vi "CSMP-Broadcast.vi"(0 "State":string, 1 "Args":string, 2 "Source/target":string, 4 "Response For Message.’Error":errorcluster, 5 "Error In":errorcluster caption="error in (no error)", 8 "Module Name":string, 10 "Msg Type":T1=enum."Broadcast(-><status>)") -> (14 "State Out":string, 15 "Args Out":string, 16 "Source/target Out":string, 17 "Pre-State Out":string, 18 "Pre-Args Out":string, 19 "Error":errorcluster)   [LabVIEW 2017, in "Communicable State Machine.lvlib"]
doc: "### CSMP-Broadcast.vi\n\n-- <b>Controls</b> --\n- <b>state</b>:\n- <b>args</b>:\n- <b>source/target</b>:\n- <b>Module Name</b>:\n- <b>Msg Type</b>:\n\n-- <b>Indicators</b> --\n- <b>state out</b>:\n- <b>args out</b>:\n- <b>source/target out</b>:\n- <b>Pre-State out</b>:\n- <b>Pre-Args out</b>:\n- <b>error</b>:"
uses:
  Communicable State Machine.lvlib
  Typedef/_CSM_MSG_TYPE.ctl
  Typedef/_CSM Status Change Event Data.ctl
  Typedef/_Cross CSM State Data.ctl
  Typedef/_Cross CSM State Response.ctl
  Typedef/_CSM_Response Source Message.ctl
  AdvanceAPI/CSM - Make String Arguments Safe.vi
  Priority Queue/Enqueue Element.vi
  ChangeFlag/FlagInstance-CSMQ FGV.vi
  ChangeFlag/FlagInstance-Broadcast Cache.vi
  _Shared/Trim Single-line Text.vi
  AdvanceAPI/CSM - Keywords.vi
  ChangeFlag/ChangeFlag-Read.vi
  CSMQ/_CSMOFGV(lvlibp).vi
  FGV-BroadcastRegistry/FGV-BroadcastRegistry(lvlibp).vi
  BroadcastRegistry/HelperVI/Broadcast Item Key.vi
  ChangeFlag/ChangeFlagDB.vi
  AdvanceAPI/CSM - List Modules.vi
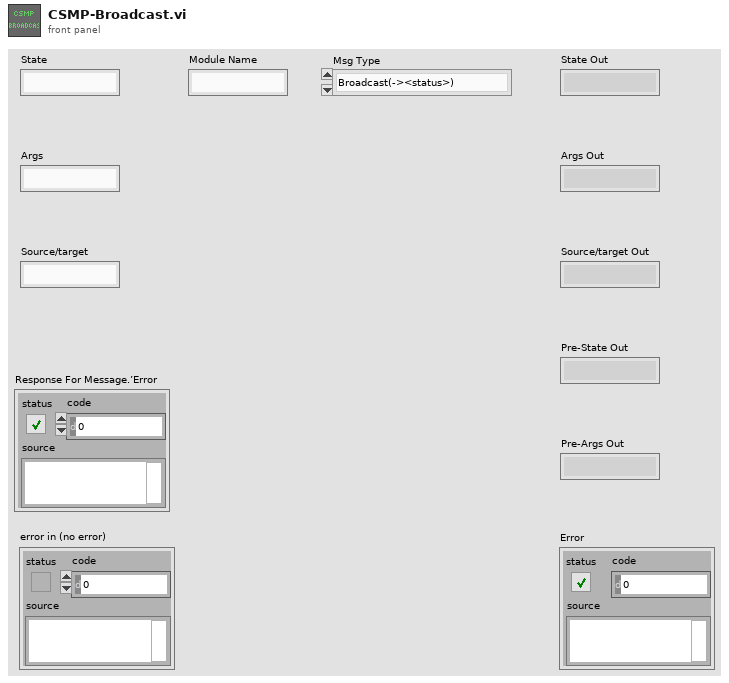
[diagram p1: front panel]
types:
  T1 = typedef "Communicable State Machine.lvlib/_CSM_MSG_TYPE.ctl" = enum16{"Sync Message(-@)", "Async Message(->)", "Async without Response(->|)", "Async Response", "Broadcast(-><all>)", "Broadcast(-><status>)", "Broadcast(-><interrupt>)", "Append to JKISM States", "Append to JKISM States(High Priority)", "Broadcast(-><state>)", "<None>"}
  T2 = typedef "Communicable State Machine.lvlib/_CSM Status Change Event Data.ctl" = cluster{"ModuleName":string, "Status":string, "Arguments":string}
  T3 = typedef "Communicable State Machine.lvlib/CSM - Broadcast Message Type.ctl" = enum16{"<Null>", "Status", "Interrupt"}
  T4 = cluster{"Target CSM":string, "Target State":string, "Register Type":T3}[]
  T5 = typedef "Communicable State Machine.lvlib/_Cross CSM State Data.ctl" = cluster{"Msg Type":T1, "state":string, "args":string, "source":string, "RespQ":refnum<queue>, "Response For Message":T6, "Target":string}
  T6 = typedef "Communicable State Machine.lvlib/_CSM_Response Source Message.ctl" = cluster{"‘State":string, "’Arguments":string, "’Error":errorcluster}
  T7 = typedef "Communicable State Machine.lvlib/_CSMObj.ctl" = cluster{"info":T8, "Refs":T10}
  T8 = typedef "Communicable State Machine.lvlib/_CSMObj-Info.ctl" = cluster{"Module Name":string, "Requested Name":string, "Group Name":string, "Mode":T9, "Allowed Messages":string[]}
  T9 = typedef "Communicable State Machine.lvlib/_CSM_MODE.ctl" = enum16{"Not Exist", "Stand Alone", "CSM", "Worker", "Worker Agent", "Chain Node", "Chain"}
  T10 = typedef "Communicable State Machine.lvlib/_CSMObj-Refs.ctl" = cluster{"WatchDogQ":refnum<queue>, "CSMDataDVR":refnum<data-value>, "Queue":T11, "GroupDataDVR":refnum<data-value>, "TagMap":refnum<data-value>, "ExitEvent":refnum<user-event>, "NewStateEvent":refnum<user-event>, "StatusEvent":refnum<user-event>, "InterruptEvent":refnum<user-event>}
  T11 = typedef "Communicable State Machine.lvlib/Priority Queue.ctl" = cluster{"HPriorityQ":refnum<queue>, "LowPriorityQ":refnum<queue>}
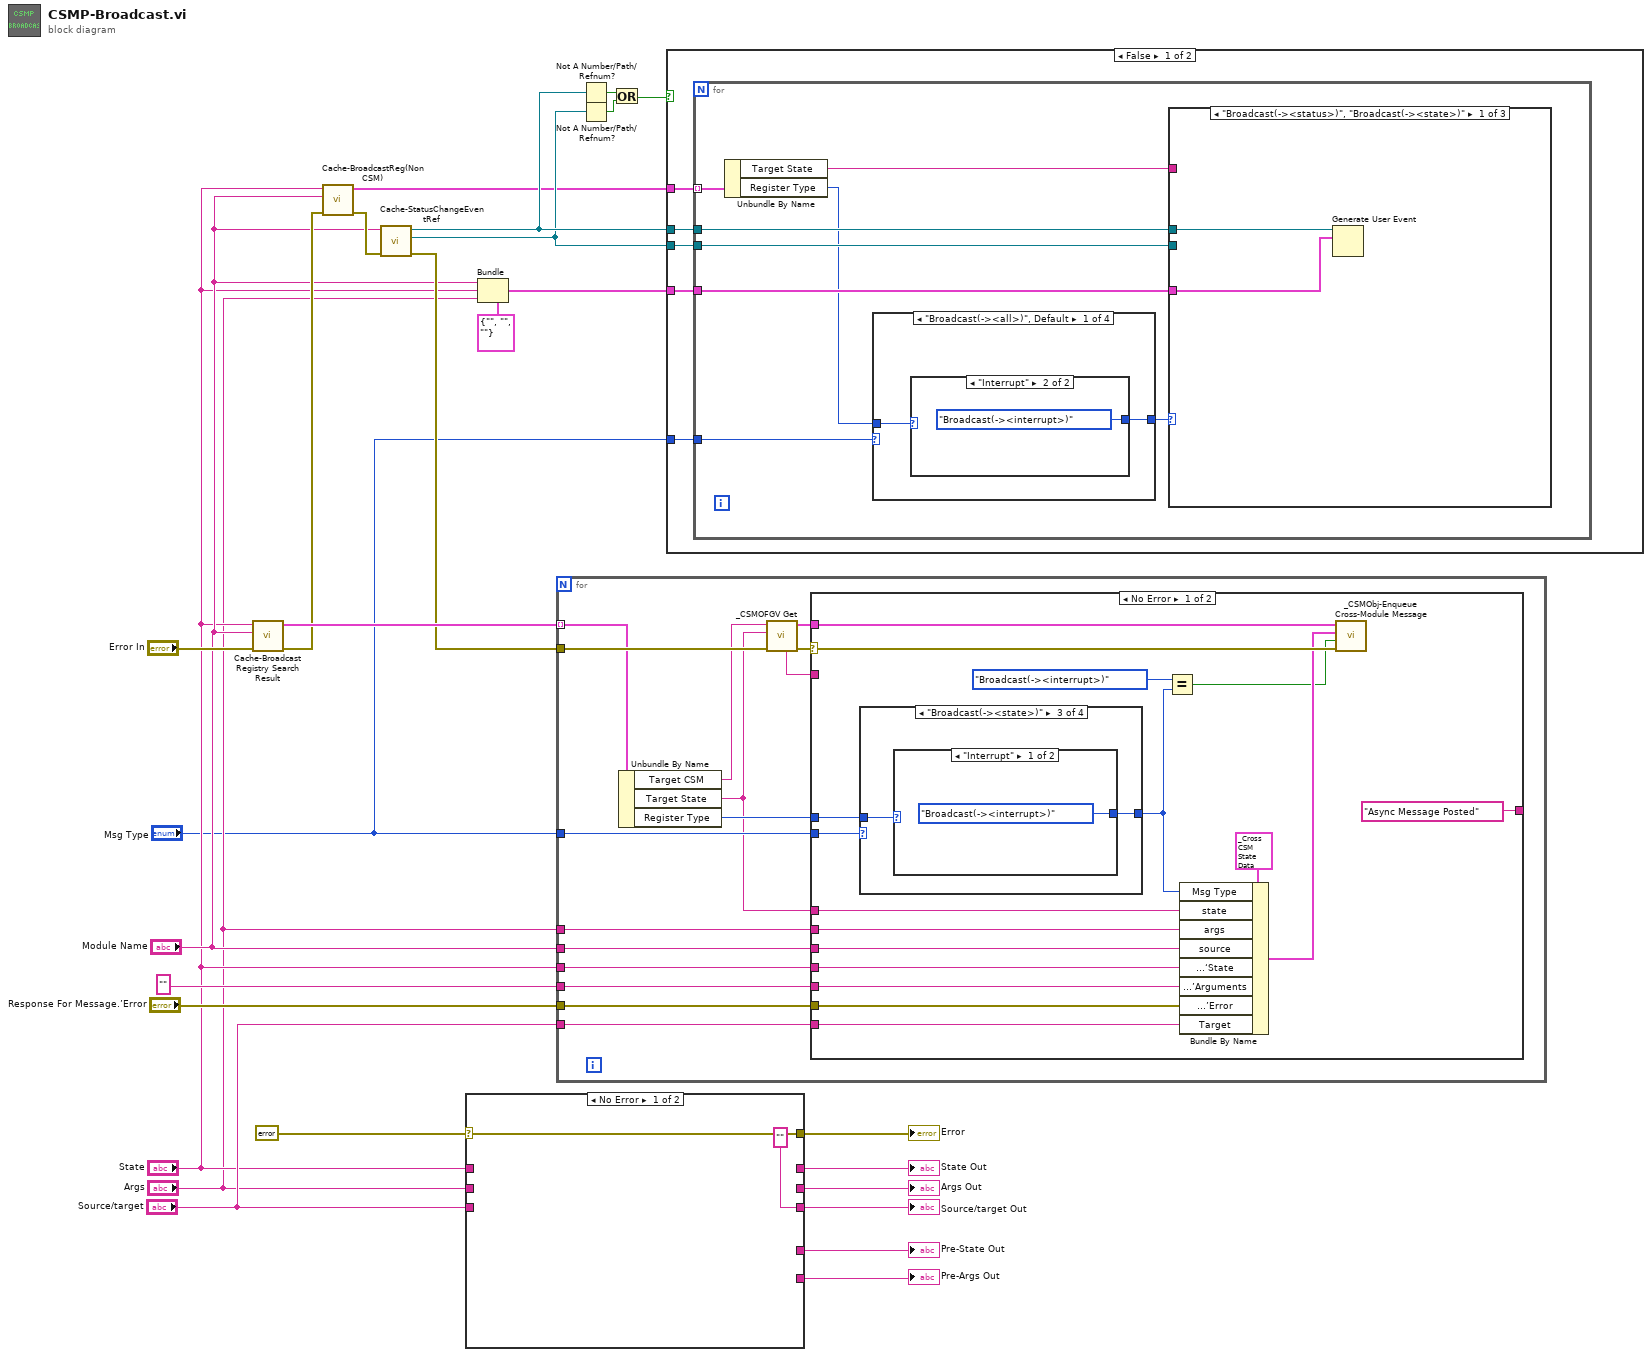
[diagram p0: block diagram]
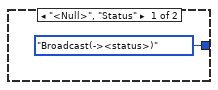
[diagram p2: hidden frame]
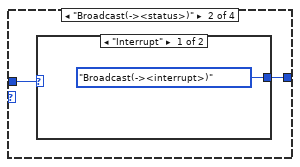
[diagram p3: hidden frame]
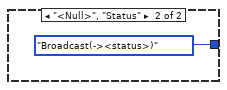
[diagram p4: hidden frame]
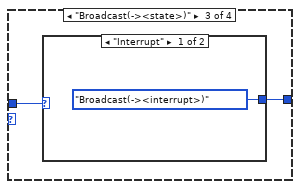
[diagram p5: hidden frame]
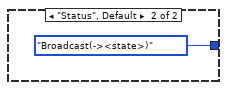
[diagram p6: hidden frame]
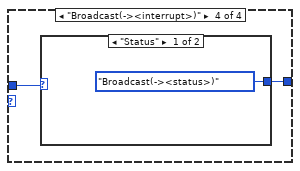
[diagram p7: hidden frame]
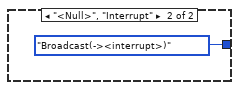
[diagram p8: hidden frame]
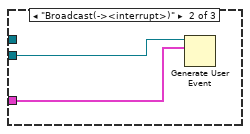
[diagram p9: hidden frame]
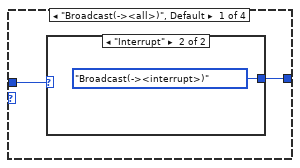
[diagram p12: hidden frame]
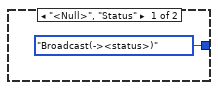
[diagram p13: hidden frame]
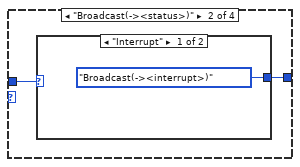
[diagram p14: hidden frame]
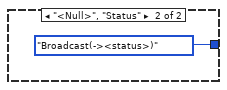
[diagram p15: hidden frame]
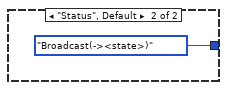
[diagram p16: hidden frame]
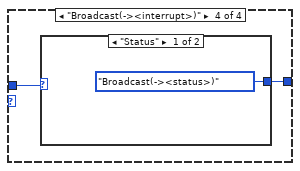
[diagram p17: hidden frame]
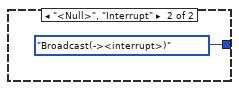
[diagram p18: hidden frame]
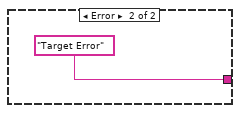
[diagram p19: hidden frame]
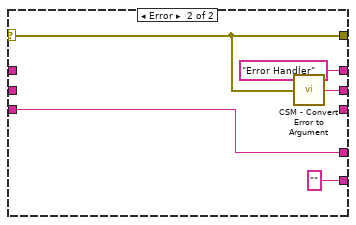
[diagram p20: hidden frame]
diagram:
  n1 = call "Cache-Broadcast Registry Search Result.vi"("error in (no error)"="Error In", "CSM Name"="Module Name", "Broadcast State"="State") -> ("error out"=w12:errorcluster, "Array"=w21:T4)  [unwired: 7 in]
  n2 = call "Cache-BroadcastReg(NonCSM).vi"("error in (no error)"=w12, "CSM Name"="Module Name", "Broadcast State"="State") -> ("error out"=w8:errorcluster, "Array"=w2:T4)  [unwired: 7 in]
  n3 = call "Cache-StatusChangeEventRef.vi"("error in (no error)"=w8, "Name (\"\" to Use UUID) In"="Module Name") -> ("error out"=w7:errorcluster, "Interrupt Event"=w6:refnum<user-event>, "Status Event"=w13:refnum<user-event>)  [unwired: 7 in]
  n4 = case shown="No Error" errorcluster {"status"=FALSE, "code"=0, "source"=""} ("error IO") {
    selector: errorcluster {"status"=FALSE, "code"=0, "source"=""} ("error IO") -> [w29 w32]
    tunnel: [_ w30] -> w27
    tunnel: [w29 w32] -> w26
    tunnel: [_ "" ("Pre-State out")] -> w25
    tunnel: "State" -> [_ _]
    tunnel: [_ "Error Handler" ("state")] -> w24
    tunnel: "Args" -> [_ _]
    tunnel: [_ w31] -> w23
    tunnel: "Source/target" -> [_ w30]
    tunnel: ["" ("source/target") _] -> w22
    frame No Error {
    }
    frame Error {
      n5 = call "CSM - Convert Error to Argument.vi"("Error"=w32) -> ("Argument"=w31:string)  [unwired: 4 in]
    }
  }
  "State Out" <- w24
  "Args Out" <- w23
  "Source/target Out" <- w22
  "Pre-State Out" <- w27
  "Pre-Args Out" <- w25
  "Error" <- w26
  n6 = Bundle(cluster=T2 {"ModuleName"="", "Status"="", "Arguments"=""} ("event data"), "ModuleName"="Module Name", "Status"="State", "Arguments"="Args") -> (w14:T2)
  n7 = for {
    tunnel: w7 -> [w46]
    tunnel: w21 -> [w42] mode=indexing
    tunnel: "Args" -> [w45]
    tunnel: "Module Name" -> [w44]
    tunnel: "State" -> [w43]
    tunnel: "Msg Type" -> [w40]
    tunnel: "Response For Message.’Error" -> [w37]
    tunnel: "" ("Response For Message.’Arguments") -> [w36]
    tunnel: "Source/target" -> [w35]
    n8 = Unbundle By Name(w42) -> ("Target CSM"=w41:string, "Target State"=w38:string, "Register Type"=w39:T3)
    n9 = call "_CSMOFGV Get.vi"("Error In"=w46, "Message"=w38, "Name (\"\" to Use UUID) In"=w41) -> ("error out"=w48:errorcluster, "CSM-Obj"=w49:T7, "Name"=w47:string)  [unwired: 6 in]
    n10 = case shown="No Error" w48 {
      selector: w48 -> [w65 _]
      tunnel: w49 -> [w66 _]
      tunnel: ["Async Message Posted" ("before match") "Target Error" ("before match")] -> _
      tunnel: w38 -> [w60 _]
      tunnel: w45 -> [w63 _]
      tunnel: w44 -> [w62 _]
      tunnel: w47 -> [_ _]
      tunnel: w43 -> [w59 _]
      tunnel: w40 -> [w54 _]
      tunnel: w39 -> [w56 _]
      tunnel: w37 -> [w52 _]
      tunnel: w36 -> [w51 _]
      tunnel: w35 -> [w50 _]
      frame No Error {
        n11 = case shown="\"Broadcast(-><state>)\"" w54 {
          tunnel: w56 -> [w68 w71 w75 w79]
          tunnel: [w67 w72 w76 w80] -> w55
          frame "Broadcast(-><all>)", Default {
            n12 = case shown="\"Interrupt\"" w68 {
              tunnel: [_CSM_MSG_TYPE."Broadcast(-><status>)" ("Msg Type") _CSM_MSG_TYPE."Broadcast(-><interrupt>)" ("Msg Type")] -> w67
              frame "<Null>", "Status" {
              }
              frame "Interrupt" {
              }
            }
          }
          frame "Broadcast(-><status>)" {
            n13 = case shown="\"Interrupt\"" w71 {
              tunnel: [_CSM_MSG_TYPE."Broadcast(-><interrupt>)" ("Msg Type") _CSM_MSG_TYPE."Broadcast(-><status>)" ("Msg Type")] -> w72
              frame "Interrupt" {
              }
              frame "<Null>", "Status" {
              }
            }
          }
          frame "Broadcast(-><state>)" {
            n14 = case shown="\"Interrupt\"" w75 {
              tunnel: [_CSM_MSG_TYPE."Broadcast(-><interrupt>)" ("Msg Type") _CSM_MSG_TYPE."Broadcast(-><state>)" ("Msg Type")] -> w76
              frame "Interrupt" {
              }
              frame "Status", Default {
              }
            }
          }
          frame "Broadcast(-><interrupt>)" {
            n15 = case shown="\"Status\"" w79 {
              tunnel: [_CSM_MSG_TYPE."Broadcast(-><status>)" ("Msg Type") _CSM_MSG_TYPE."Broadcast(-><interrupt>)" ("Msg Type")] -> w80
              frame "Status" {
              }
              frame "<Null>", "Interrupt" {
              }
            }
          }
        }
        n16 = Equal?(x=_CSM_MSG_TYPE."Broadcast(-><interrupt>)", y=w55) -> (x = y?=w57:bool)
        n17 = Bundle By Name(cluster=T5 {"Msg Type"=enum."Sync Message(-@)", "state"="", "args"="", "source"="", "RespQ"=refnum, "Response For Message"={"‘State"="", "’Arguments"="", "’Error"={"status"=FALSE, "code"=0, "source"=""}}, "Target"=""} ("Cross JKI State Machine State"), "Msg Type"=w55, "state"=w60, "args"=w63, "source"=w62, "Response For Message.‘State"=w59, "Response For Message.’Arguments"=w51, "Response For Message.’Error"=w52, "Target"=w50) -> (w61:T5)
        n18 = call "_CSMObj-Enqueue Cross-Module Message.vi"("Error In"=w65, "High Priority? (F)"=w57, "Data"=w61, "CSMQ In"=w66) -> ()  [unwired: 6 in, 2 out]
      }
      frame Error {
      }
    }
  }
  n19 = Not A Number/Path/Refnum?(number/path/refnum=w13) -> (NaN/Path/Refnum?=w10:bool)
  n20 = Not A Number/Path/Refnum?(number/path/refnum=w6) -> (NaN/Path/Refnum?=w9:bool)
  n21 = Or(x=w10, y=w9) -> (x .or. y?=w11:bool)
  n22 = case shown="False" w11 {
    tunnel: w13 -> [w88 _]
    tunnel: w14 -> [w87 _]
    tunnel: w6 -> [w85 _]
    tunnel: w2 -> [w86 _]
    tunnel: "Msg Type" -> [w84 _]
    frame False {
      n23 = for {
        tunnel: w88 -> [w96]
        tunnel: w87 -> [w95]
        tunnel: w86 -> [w94] mode=indexing
        tunnel: w85 -> [w93]
        tunnel: w84 -> [w91]
        n24 = Unbundle By Name(w94) -> ("Target State"=w92:string, "Register Type"=w90:T3)
        n25 = case shown="\"Broadcast(-><all>)\", Default" w91 {
          tunnel: w90 -> [w98 w101 w105 w109]
          tunnel: [w97 w102 w106 w110] -> w89
          frame "Broadcast(-><all>)", Default {
            n26 = case shown="\"Interrupt\"" w98 {
              tunnel: [_CSM_MSG_TYPE."Broadcast(-><status>)" ("Msg Type") _CSM_MSG_TYPE."Broadcast(-><interrupt>)" ("Msg Type")] -> w97
              frame "<Null>", "Status" {
              }
              frame "Interrupt" {
              }
            }
          }
          frame "Broadcast(-><status>)" {
            n27 = case shown="\"Interrupt\"" w101 {
              tunnel: [_CSM_MSG_TYPE."Broadcast(-><interrupt>)" ("Msg Type") _CSM_MSG_TYPE."Broadcast(-><status>)" ("Msg Type")] -> w102
              frame "Interrupt" {
              }
              frame "<Null>", "Status" {
              }
            }
          }
          frame "Broadcast(-><state>)" {
            n28 = case shown="\"Interrupt\"" w105 {
              tunnel: [_CSM_MSG_TYPE."Broadcast(-><interrupt>)" ("Msg Type") _CSM_MSG_TYPE."Broadcast(-><state>)" ("Msg Type")] -> w106
              frame "Interrupt" {
              }
              frame "Status", Default {
              }
            }
          }
          frame "Broadcast(-><interrupt>)" {
            n29 = case shown="\"Status\"" w109 {
              tunnel: [_CSM_MSG_TYPE."Broadcast(-><status>)" ("Msg Type") _CSM_MSG_TYPE."Broadcast(-><interrupt>)" ("Msg Type")] -> w110
              frame "Status" {
              }
              frame "<Null>", "Interrupt" {
              }
            }
          }
        }
        n30 = case shown="\"Broadcast(-><status>)\", \"Broadcast(-><state>)\"" w89 {
          tunnel: w96 -> [w114 _ _]
          tunnel: w95 -> [w113 w116 _]
          tunnel: w93 -> [_ w115 _]
          tunnel: w92 -> [_ _ _]
          frame "Broadcast(-><status>)", "Broadcast(-><state>)" {
            n31 = Generate User Event(user event=w114, event data cluster=w113) -> ()  [unwired: 2 in, 2 out]
          }
          frame "Broadcast(-><interrupt>)" {
            n32 = Generate User Event(user event=w115, event data cluster=w116) -> ()  [unwired: 2 in, 2 out]
          }
          frame Default {
          }
        }
      }
    }
    frame True {
    }
  }
